vi "1_1_Periodic Sampling-Baseband signal.vi"() -> ()   [LabVIEW 2009]
uses:
  <vilib>/measure/maspectr.llb/FFT Power Spectrum for 1 Chan.vi
  <vilib>/measure/matone.llb/Extract Single Tone Information 1 Chan.vi
  <vilib>/Analysis/2dsp.llb/Power Spectrum (DBL).vi
  <vilib>/measure/NI_MAPro.lvlib
  <vilib>/Analysis/NI_AALPro.lvlib
panel:
  out "?":string="Linear "
  in  "Window":T1(ring)
  out "Nyquist Freq":dbl=500.0
  in  "phase":dbl format="%.2f"
  out "Power Spectrum 2 : using Direct\nPower spectrum vi. No window is\napplied to this.":cluster{dbl, dbl, "Power Spectrum":dbl[]}(graph)={-490.0, 10.0, "Power Spectrum"=[6.8644289717974e-06, 6.948348866432592e-06, 7.090512711300904e-06, 7.294482758807924e-06, 7.565488211844803e-06, 7.910690881066599e-06, 8.339563748447707e-06, 8.864416556071993e-06, 9.501118610394658e-06, 1.027009254666942e-05, 1.1197688183637622e-05, 1.2318099949098075e-05, 1.3676076667737237e-05, 1.533080945009513e-05, 1.7361608610958907e-05, 1.9876360694174385e-05, 2.302441736444572e-05, 2.7016754139611615e-05, 3.215844634250416e-05, 3.8902800543660375e-05, 4.7945223887713574e-05, 6.039375965804807e-05, 7.809661448434991e-05, 0.00010431520530875186, 0.00014522871546541753, 0.0002136813008334414, 0.0003399668131708884, 0.0006099526244035307, 0.0013511776127591581, 0.004819311031301696, 0.22363965046951875, 0.01075042966426908, 0.002299457774904508, 0.0010080590440551206, 0.0005790679243009003, 0.00038415924500042735, 0.00027891999235177815, 0.00021553252750768868, 0.00017438855462520583, 0.0001462170132831988, 0.0001261636134395579, 0.00011148460530840962, 0.00010053512956452468, 9.22831439253106e-05, 8.605849437347107e-05, 8.141575174439822e-05, 7.805581046861667e-05, 7.577964197441328e-05, 7.44606535237127e-05, 7.402851164525869e-05, 7.44606535237127e-05, 7.577964197441328e-05, 7.805581046861667e-05, 8.141575174439822e-05, 8.605849437347107e-05, 9.22831439253106e-05, 0.00010053512956452468, 0.00011148460530840962, 0.0001261636134395579, 0.0001462170132831988, 0.00017438855462520583, 0.00021553252750768868, 0.00027891999235177815, 0.00038415924500042735, 0.0005790679243009003, 0.0010080590440551206, 0.002299457774904508, 0.01075042966426908, 0.22363965046951875, 0.004819311031301696, 0.0013511776127591581, 0.0006099526244035307, 0.0003399668131708884, 0.0002136813008334414, 0.00014522871546541753, 0.00010431520530875186, 7.809661448434991e-05, 6.039375965804807e-05, 4.7945223887713574e-05, 3.8902800543660375e-05, 3.215844634250416e-05, 2.7016754139611615e-05, 2.302441736444572e-05, 1.9876360694174385e-05, 1.7361608610958907e-05, 1.533080945009513e-05, 1.3676076667737237e-05, 1.2318099949098075e-05, 1.1197688183637622e-05, 1.027009254666942e-05, 9.501118610394658e-06, 8.864416556071993e-06, 8.339563748447707e-06, 7.910690881066599e-06, 7.565488211844803e-06, 7.294482758807924e-06, 7.090512711300904e-06, 6.948348866432592e-06, 6.8644289717974e-06, 6.83668216211769e-06]}
  out "Detected phase (deg)":dbl=8.750949106683947e-06 format="%.2p"
  out "Detected amplitude":dbl=0.9999999964821926 format="%.2p"
  out "Detected frequency":dbl=188.23506603488084 format="%.2p"
  in  "stop":bool
  in  "?":bool
  out "Power Spectrum: Using FFT Power \nspectrum express vi.":cluster{"f0":dbl, "df":dbl, "magnitude":dbl[]}(graph)={"f0"=0.0, "df"=10.0, "magnitude"=[7.402851164525869e-05, 0.0001489213070474254, 0.00015155928394882656, 0.00015611162093723334, 0.00016283150348879644, 0.00017211698874694214, 0.0001845662878506212, 0.00020107025912904935, 0.00022296921061681923, 0.0002523272268791158, 0.0002924340265663976, 0.00034877710925041165, 0.00043106505501537735, 0.0005578399847035563, 0.0007683184900008547, 0.0011581358486018006, 0.0020161180881102412, 0.004598915549809016, 0.02150085932853816, 0.4472793009390375, 0.009638622062603392, 0.0027023552255183163, 0.0012199052488070614, 0.0006799336263417768, 0.0004273626016668828, 0.00029045743093083506, 0.00020863041061750372, 0.00015619322896869982, 0.00012078751931609614, 9.589044777542715e-05, 7.780560108732075e-05, 6.431689268500832e-05, 5.403350827922323e-05, 4.604883472889144e-05, 3.975272138834877e-05, 3.4723217221917814e-05, 3.066161890019026e-05, 2.7352153335474473e-05, 2.463619989819615e-05, 2.2395376367275244e-05, 2.054018509333884e-05, 1.9002237220789316e-05, 1.7728833112143987e-05, 1.6679127496895414e-05, 1.5821381762133197e-05, 1.5130976423689606e-05, 1.4588965517615849e-05, 1.4181025422601809e-05, 1.3896697732865183e-05, 1.37288579435948e-05]}
  in  "Fs":dbl=1000.0
  in  "Signal Frequency":dbl(knob)=188.23506637766508 scale=0.0..5000.0
  in  "Amplitude":dbl(knob)=1.0 scale=0.0..10.0
  in  "#s":i32=100
  in  "Reset phase":bool=TRUE
  out "Signal waveform":waveform(dbl)(graph)={"t0"=timestamp(0 s since 1904-01-01), "dt"=0.001, "Y"=[0.0, 0.9256371182999356, 0.7005450798463589, -0.395447263988239, -0.9998293562099383, -0.3612483377020396, 0.7264276736535595, 0.9110267795788056, -0.036940059744579944, -0.938983931027988, -0.6737062182964252, 0.42910639137585854, 0.9984645553012055, 0.3265562952090511, -0.7513186691015249, -0.8951728584714161, 0.0738296950574357, 0.9510489989118901, 0.6459477249580868, -0.4621797740168831, -0.9957368164831695, -0.29141849232136374, 0.7751840891390788, 0.8780969961166252, -0.11061855033789693, -0.961815852725658, -0.6173074911141917, 0.49462226562469264, 0.991649863211633, 0.2558828933291016, -0.7979913566601833, -0.8598225016444524, 0.14725640755345615, 0.9712697953494527, 0.5878246116532049, -0.5263895811002975, -0.9862092743161239, -0.21999800552750523, 0.8197093389728166, 0.8403743203583028, -0.18369325478909213, -0.9793979218316428, -0.5575393317033808, 0.5574383569829624, 0.9794224763846116, 0.18381281300290128, -0.8403083902960987, -0.8197789996838377, 0.21987935451515805, 0.9861891370044908, 0.5264929916968198, -0.5877262106428011, -0.9712987336259616, -0.14737670976771916, 0.8597603922278314, 0.7980646529307909, -0.25576531148087145, -0.9916341706294493, -0.4947279709383411, 0.6172117981345275, 0.9618491352239736, 0.11073943233600023, -0.8780387921270546, -0.7752609209173702, 0.29130214014046785, 0.9957255900513411, 0.46228762975631943, -0.6458548706333203, -0.9510865802002743, -0.07395099183134876, 0.8951186393593124, 0.7513989315095172, -0.32644133152015925, -0.9984578103441903, -0.42921625031434213, 0.6736163293758551, 0.9390257598067064, 0.03706160572010313, -0.9109766193550908, -0.7265112571303465, 0.361134919434479, 0.9998271019348288, 0.39555897616459845, -0.7004582790314036, -0.9256831374712873, -0.00012162926276310762, 0.9255910854350092, 0.7006318702976664, -0.3953355459617792, -0.999831595693894, -0.36136175062537546, 0.7263440794302658, 0.9110769263250629, -0.03681851322263691, -0.9389420883582673, -0.6737960972503468, 0.4289965260893886, 0.9984712854872528, 0.32667125406688063, -0.7512383955788371]}
  # "Periodic Sampling and Aliasing single tone."
  # "SIGNAL INFORMATION"
  # "DETECTED SIGNAL INFORMATION"
  # "SAMPLING INFORMATION"
  # "Program Developed by Indranil Sinharoy"
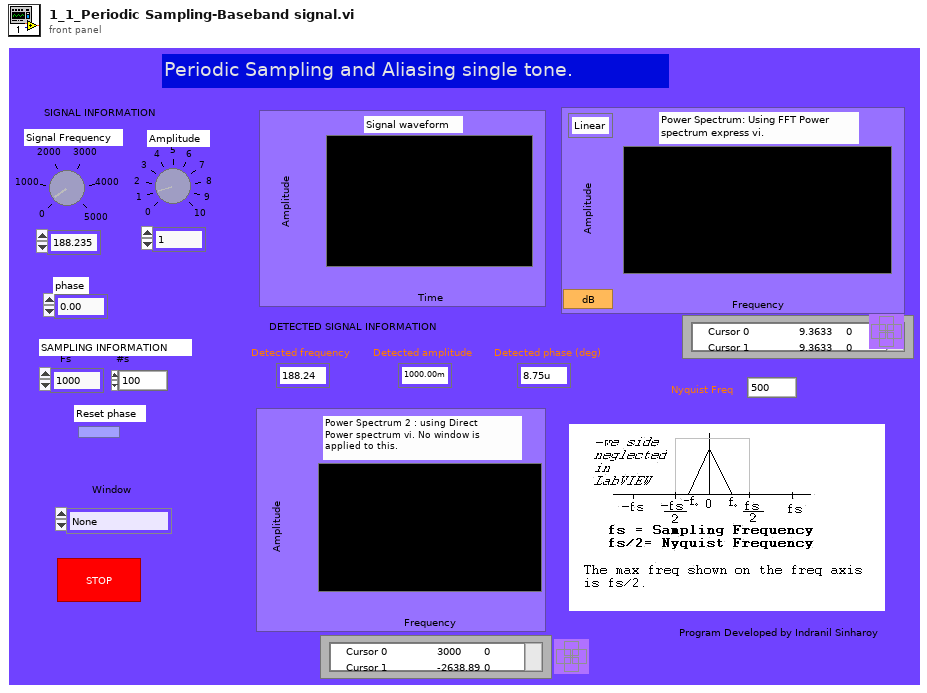
[diagram p1: front panel]
types:
  T1 = enum16{"None ", "Hanning", "Hamming", "Blackman-Harris", "Exact Blackman", "Blackman", "Flat Top", "4 Term B-Harris ", "7 Term B-Harris", "Low Sidelobe"}
  T2 = cluster{dbl, "fundamental frequency":dbl, "reversed array":cdb[]}
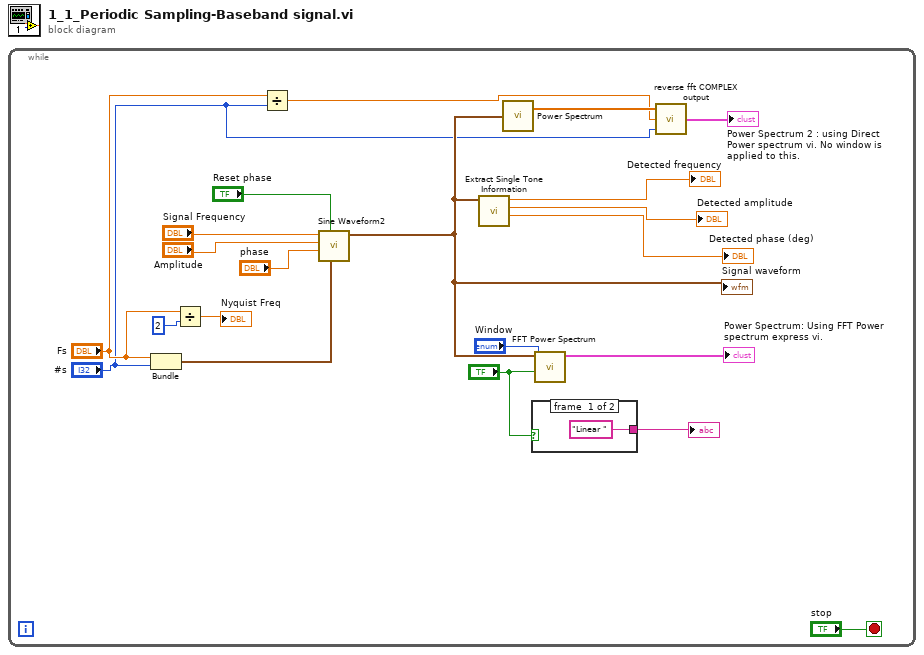
[diagram p0: block diagram]
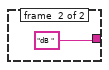
[diagram p2: hidden frame]
diagram:
  n1 = while {
    stop <- "stop" stop-if-true
    n2 = Bundle("Fs"="Fs", "#s"="#s") -> (w11:cluster{"Fs":dbl, "#s":i32})  [unwired: 1 in]
    n3 = Divide(x="Fs", y=2) -> (x/y=→"Nyquist Freq":dbl)
    n4 = Divide(x="Fs", y="#s") -> (x/y=w3:dbl)
    n5 = call "Sine Waveform2.vi"("sampling info"=w11, "reset signal"="Reset phase", "phase"="phase", "amplitude"="Amplitude", "frequency"="Signal Frequency") -> ("signal out"=w16:waveform(dbl))  [unwired: 5 in, 1 out]
    "Signal waveform" <- w16
    n6 = call-poly <vilib>:"Extract Single Tone Information.vi"("time signal in"=w16) -> ("detected phase (deg)"=→"Detected phase (deg)":dbl, "detected amplitude"=→"Detected amplitude":dbl, "detected frequency"=→"Detected frequency":dbl)  [unwired: 5 in, 3 out]
    n7 = call-poly <vilib>:"Power Spectrum.vi"("X"=w16) -> ("Power Spectrum"=w4:dbl[])  [unwired: 1 out]
    n8 = case shown="True" "?" {
      tunnel: ["Linear " "dB "] -> w5
      frame #0 {
      }
      frame #1 {
      }
    }
    "?" <- w5
    n9 = call-poly <vilib>:"FFT Power Spectrum.vi"("dB On (F)"="?", "window"="Window", "time signal"=w16) -> ("power spectrum"=→"Power Spectrum: Using FFT Power \nspectrum express vi.":cluster{"f0":dbl, "df":dbl, "magnitude":dbl[]})  [unwired: 5 in, 3 out]
    n10 = call "reverse fft COMPLEX output.vi"("samples"="#s", "fundamental frequency"=w3, "fft output"=w4) -> ("Reversed FFT COMPLEX O/P"=→"Power Spectrum 2 : using Direct\nPower spectrum vi. No window is\napplied to this.":T2)
  }
